vi "libssh2_channel_read_ex.vi"(8 "error in (no error)":errorcluster, 9 "buffer length":i32=1024, 10 "stream id":i32, 11 "channel":T1) -> (0 "error out":errorcluster, 2 "buffer":u8[](array[numeric]))   [LabVIEW 2013, in "libssh2.lvlib"]
doc: "Read data from a channel.\nAll channel streams have one standard input/output substream (<B>stream id</B> = 0), and may have up to 2^32 extended data streams as identified by the selected <B>stream id</B>. The SSH-2 protocol currently defines a standard stream ID of 1 to be the stderr substream."
uses:
  libssh2.lvlib
  Channel Refnum.ctl
  Not A Channel.vi
  <vilib>/Utility/error.llb/Error Cluster From Error Code.vi
  Global Settings.vi
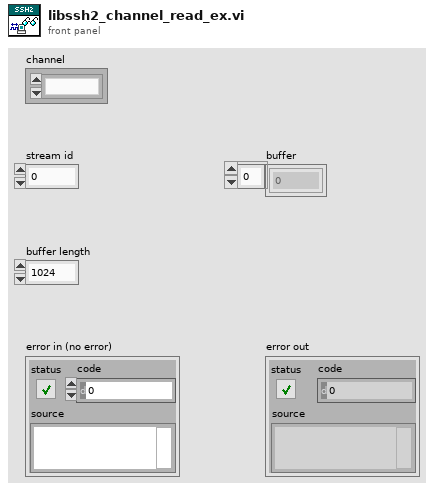
[diagram p1: front panel]
types:
  T1 = typedef "libssh2.lvlib/Channel Refnum.ctl" = refnum<k1>
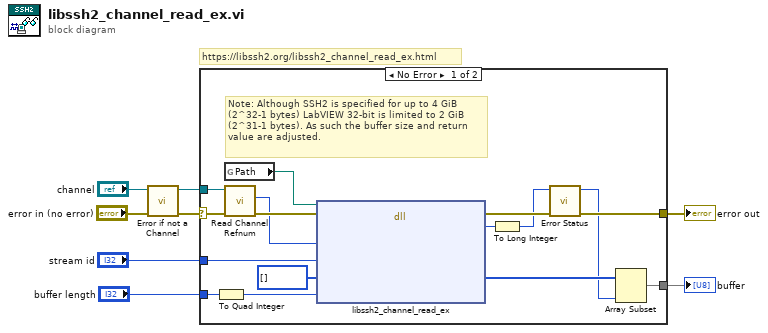
[diagram p0: block diagram]
diagram:
  # "https://libssh2.org/libssh2_channel_read_ex.html"
  n1 = call "Error if not a Channel.vi"("error in (no error)"="error in (no error)", "channel"="channel") -> ("error out"=w3:errorcluster, "channel out"=w1:T1)  [unwired: 8 in]
  n2 = case shown="No Error" w3 {
    selector: w3 -> [w21 w25]
    tunnel: "stream id" -> [w24 _]
    tunnel: "buffer length" -> [w23 _]
    tunnel: [w20 w25] -> w6
    tunnel: [w22 _] -> w5
    tunnel: w1 -> [w19 _]
    frame No Error {
      # "Note: Although SSH2 is specified for up to 4 GiB\n(2^32-1 bytes) LabVIEW 32-bit is limited to 2 GiB\n(2^31-1 bytes). As such the buffer size and return\nvalue are adjusted."
      n3 = To Quad Integer(1:w23) -> (0:w10:i64)
      n4 = global read "Global Settings.vi" "Path"() -> (w14:path)
      n5 = call "Read Channel Refnum.vi"("error in (no error)"=w21, "channel"=w19) -> ("error out"=w16:errorcluster, "LIBSSH2_CHANNEL*"=w15:u64)  [unwired: 8 in]
      n6 = dll-call lib="?" fn="libssh2_channel_read_ex"(path in=w14, error in=w16, "channel"=w15, "stream_id"=w24, "buf"=u8[] [], "buflen"=w10) -> (error out=w18:errorcluster, "return value"=w13:i64, "buf"=w17:u8[])  [unwired: 4 in, 1 out]
      n7 = To Long Integer(number=w13) -> (32bit integer=w12:i32)
      n8 = call "Error Status.vi"("error in (no error)"=w18, "return value"=w12) -> ("error out"=w20:errorcluster, "return value out"=w11:i32)  [unwired: 8 in]
      n9 = Array Subset(array=w17, length=w11) -> (w22:u8[])  [unwired: 1 in]
    }
    frame Error {
    }
  }
  "error out" <- w6
  "buffer" <- w5
